vi "SHsT(U)_ECD.vi"(7 "SpannungenSH[V]":dbl[](array[numeric]), 9 "Traps/MachKoeff2":dbl[](array[numeric]), 10 "Traps/MachKoeff1":dbl[](array[numeric]), 11 "Traps/MachKoeff0":dbl[](array[numeric])) -> (3 "TemperaturenSH[°C]":dbl[](array[numeric]))   [LabVIEW 2017]
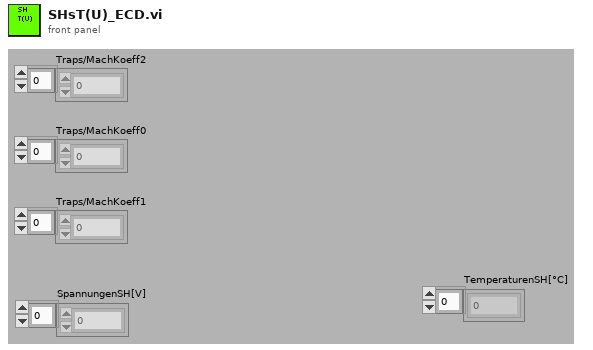
[diagram p1: front panel]
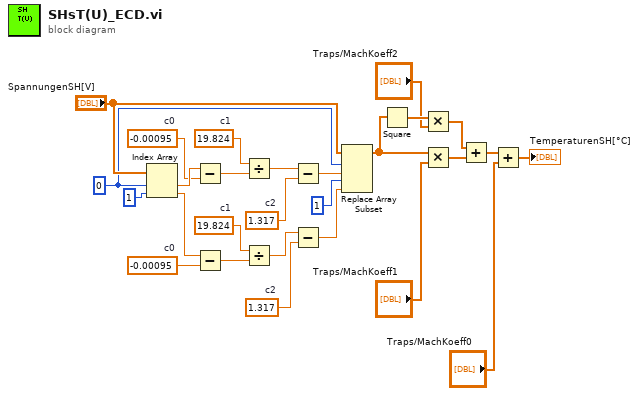
[diagram p0: block diagram]
diagram:
  w4 = 1.317  # c2
  w7 = 19.824  # c1
  w8 = -0.00095  # c0
  w11 = 1.317  # c2
  w14 = 19.824  # c1
  w15 = -0.00095  # c0
  w18 = 0 ("index")
  n1 = Index Array(array="SpannungenSH[V]", index #1=w18, index #2=1 ("index")) -> (element #1=w16:dbl, element #2=w2:dbl)
  n2 = Subtract(x=w16, y=w15) -> (x-y=w13:dbl)
  n3 = Subtract(x=w2, y=w8) -> (x-y=w6:dbl)
  n4 = Divide(x=w14, y=w13) -> (x/y=w12:dbl)
  n5 = Divide(x=w7, y=w6) -> (x/y=w5:dbl)
  n6 = Subtract(x=w12, y=w11) -> (x-y=w10:dbl)
  n7 = Subtract(x=w5, y=w4) -> (x-y=w1:dbl)
  n8 = Replace Array Subset(array="SpannungenSH[V]", new element #1=w10, index #1=w18, new element #2=w1, index #2=1 ("index")) -> (w17:dbl[])
  n9 = Square(x=w17) -> (x^2=w24:dbl[])
  n10 = Multiply(x=w24, y="Traps/MachKoeff2") -> (x*y=w25:dbl[])
  n11 = Multiply(x=w17, y="Traps/MachKoeff1") -> (x*y=w26:dbl[])
  n12 = Add(x=w25, y=w26) -> (x+y=w27:dbl[])
  n13 = Add(x=w27, y="Traps/MachKoeff0") -> (x+y=→"TemperaturenSH[°C]":dbl[])
